vi "Fail.vi"(7 "Description":string, 8 "error in (no error)":errorcluster, 9 "Message":string, 11 "LUnit Test Case In":refnum<class "LUnit Test Case V2.lvclass">) -> (0 "error out":errorcluster, 3 "LUnit Test Case Out":refnum<class "LUnit Test Case V2.lvclass">)   [LabVIEW 2020, in "LUnit Test Case V2.lvclass"]
doc: "Generates a fail result for the calling test method. A description and message may be provided."
uses:
  LUnit Test Case V2.lvclass
  LUnit Test Case V2.lvclass/LUnit Test Case V2.ctl
  Result/Status.ctl
  Result/Result.lvlib
  Result/Type.ctl
  Result/Result.ctl
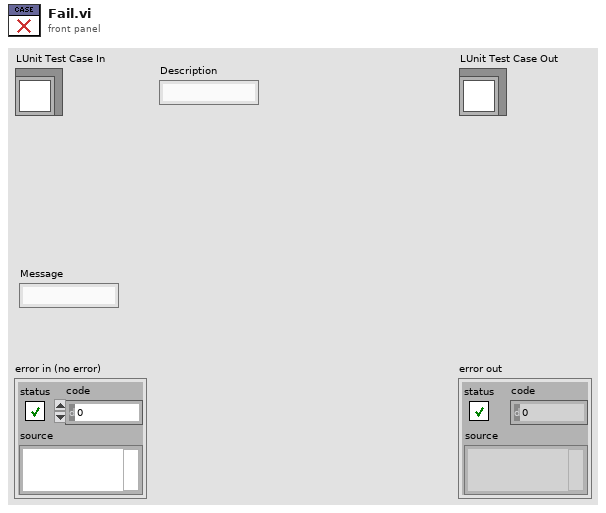
[diagram p1: front panel]
types:
  T1 = typedef "Result.lvlib/Result.ctl" = cluster{"Case":string, "Method":string, "Message":string, "Description":string, "Status":T2, "Result Type":T3}
  T2 = typedef "Result.lvlib/Status.ctl" = enum16{"Pass", "Fail", "Error", "Skipped", "Setup Error", "Broken", "Teardown Error"}
  T3 = typedef "Result.lvlib/Type.ctl" = enum16{"None", "Pass", "Fail", "Skip", "Pass if Equal", "Fail if Equal", "Pass if Error", "Fail if Error", "Pass if", "Fail if"}
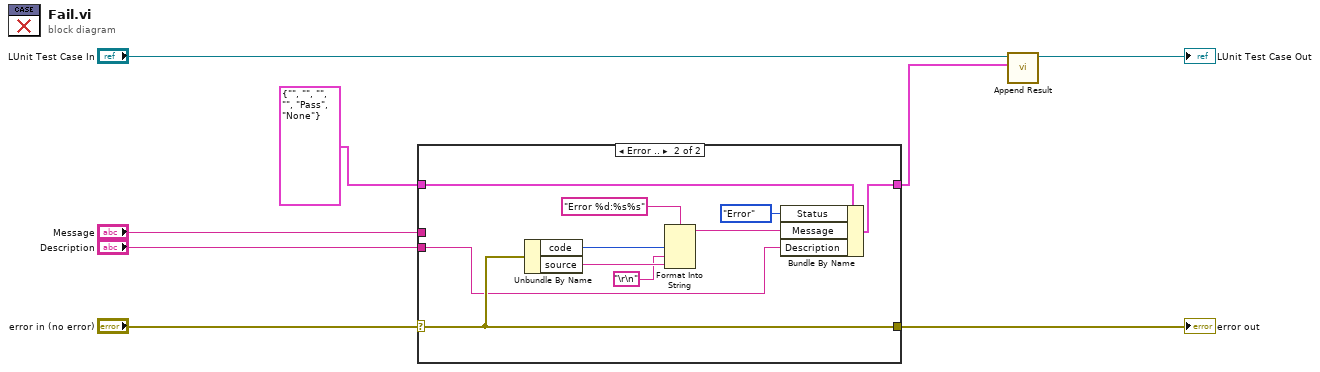
[diagram p0: block diagram]
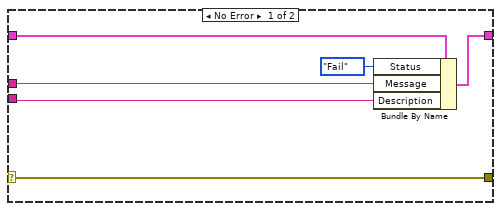
[diagram p2: hidden frame]
diagram:
  n1 = case shown="Error .." "error in (no error)" {
    selector: "error in (no error)" -> [w12 w20]
    tunnel: T1 {"Case"="", "Method"="", "Message"="", "Description"="", "Status"=enum."Pass", "Result Type"=enum."None"} ("Temporary Assertion Result") -> [w14 w17]
    tunnel: [w13 w18] -> w1
    tunnel: [w12 w20] -> w5
    tunnel: "Message" -> [w11 _]
    tunnel: "Description" -> [w10 w16]
    frame No Error {
      n2 = Bundle By Name(cluster=w14, "Status"=Status."Fail", "Message"=w11, "Description"=w10) -> (w13:T1)
    }
    frame Error {
      n3 = Unbundle By Name(w20) -> ("code"=w24:i32, "source"=w22:string)
      n4 = Format Into String(format string="Error %d:%s%s", w24, "\r\n", w22) -> (resulting string=w23:string)  [unwired: 2 in, 1 out]
      n5 = Bundle By Name(cluster=w17, "Status"=Status."Error", "Message"=w23, "Description"=w16) -> (w18:T1)
    }
  }
  "error out" <- w5
  n6 = call "Append Result.vi"("Temporary Assertion Result"=w1, "LUnit Test Case V2 in"="LUnit Test Case In") -> ("LUnit Test Case V2 out"=→"LUnit Test Case Out":refnum<class "LUnit Test Case V2.lvclass">)  [unwired: 9 in]
